vi "Tachometer.vi"(11 "Enum":enum16{"Start", "Run", "End"}(ring)) -> (3 "Tach out":dbl)   [LabVIEW 2012]
uses:
  TypeDefs/Digital Module 1.ctl
  <vilib>/Rock Robotics/SystemInterfaces/Typedef/FPGA_TypedefDigitalModule.ctl
  <vilib>/Rock Robotics/SystemInterfaces/DIO/FPGA_DIOChannel.ctl
  <vilib>/Rock Robotics/WPI/Counter/WPI_CounterDigitalInputToDigitalSource.vi
  <vilib>/Rock Robotics/WPI/Counter/WPI_CounterOpen Gear Tooth Sensor Mode.vi
panel:
  in  "Digital Module A":T1={"Module"=enum."Digital Module 1", "Unassigned"=enum."DIO 1", "Unassigned"=enum."DIO 2", "Unassigned"=enum."DIO 3", "Unassigned"=enum."DIO 4", "Unassigned"=enum."DIO 5", "Unassigned"=enum."DIO 6", "Unassigned"=enum."DIO 7", "Unassigned"=enum."DIO 8", "Unassigned"=enum."DIO 9", "Unassigned"=enum."DIO 10", "Unassigned"=enum."DIO 11", "Unassigned"=enum."DIO 12", "Unassigned"=enum."DIO 13", "Unassigned"=enum."DIO 14"}
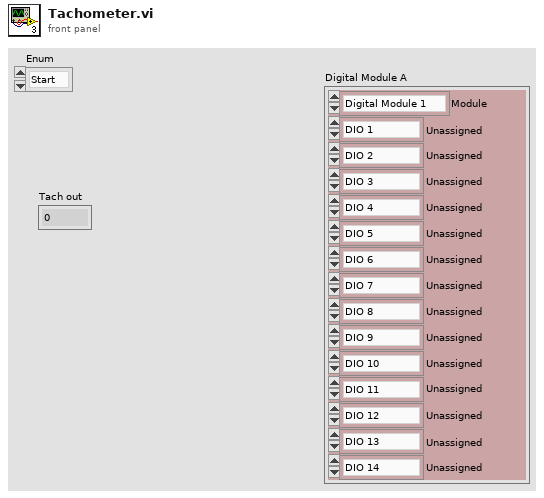
[diagram p1: front panel]
types:
  T1 = typedef "Digital Module 1.ctl" = cluster{"Module":T2, "Unassigned":T3, "Unassigned":T3, "Unassigned":T3, "Unassigned":T3, "Unassigned":T3, "Unassigned":T3, "Unassigned":T3, "Unassigned":T3, "Unassigned":T3, "Unassigned":T3, "Unassigned":T3, "Unassigned":T3, "Unassigned":T3, "Unassigned":T3}
  T2 = typedef "FPGA_TypedefDigitalModule.ctl" = enum16{"Digital Module 1", "Digital Module 2"}
  T3 = typedef "FPGA_DIOChannel.ctl" = enum8{"DIO 1", "DIO 2", "DIO 3", "DIO 4", "DIO 5", "DIO 6", "DIO 7", "DIO 8", "DIO 9", "DIO 10", "DIO 11", "DIO 12", "DIO 13", "DIO 14", "Invalid"}
  T4 = typedef "WPI_DigitalInputDevRef.ctl" = cluster{"DevStatus":errorcluster, "DIO Channel":T3, "Digital Module":T2}
  T5 = typedef "FPGA_CounterEncoderSourceConvertionLVSourceType.ctl" = cluster{"DevStatus":errorcluster, "AnalogTriggerMode?":bool, "DigitalMode":cluster{"Digital Module":T2, "DIO Channel":T6}, "AnalogTriggerMode":cluster{"AnalogTriggerIndex":T7, "OutputType":T8}}
  T6 = typedef "FPGA_DIODigitalSourceChannel.ctl" = enum8{"DIO 1", "DIO 2", "DIO 3", "DIO 4", "DIO 5", "DIO 6", "DIO 7", "DIO 8", "DIO 9", "DIO 10", "DIO 11", "DIO 12", "DIO 13", "DIO 14", "Disabled"}
  T7 = typedef "FPGA_AnalogTriggerIndex.ctl" = enum8{"Trig 0", "Trig 1", "Trig 2", "Trig 3", "Trig 4", "Trig 5", "Trig 6", "Trig 7", "Invalid"}
  T8 = typedef "FPGA_AnalogTriggerOutType.ctl" = enum16{"InWindow", "TriggerState", "Rising", "Falling"}
  T9 = typedef "WPI_CounterDevRef.ctl" = cluster{"DevStatus":errorcluster, "CntIndex":T10}
  T10 = typedef "FPGA_CounterCtrSystemIndex.ctl" = enum8{"Ctr 0", "Ctr 1", "Ctr 2", "Ctr 3", "Ctr 4", "Ctr 5", "Ctr 6", "Ctr 7", "Invalid"}
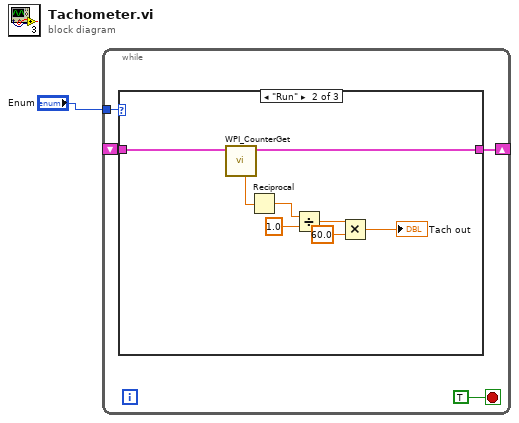
[diagram p0: block diagram]
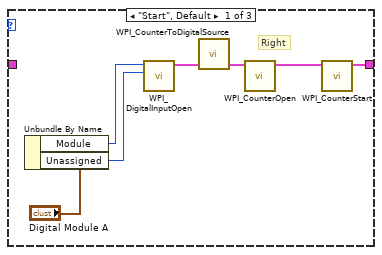
[diagram p2: hidden frame]
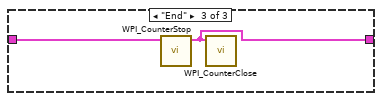
[diagram p3: hidden frame]
diagram:
  n1 = while {
    shift-right: [w4] -> _
    shift-left: _ -> [w3]
    tunnel: "Enum" -> [w2]
    stop <- TRUE stop-if-true
    n2 = case shown="\"Run\"" w2 {
      tunnel: [w8 w19 w21] -> w4
      tunnel: w3 -> [_ w20 w22]
      frame "Start", Default {
        # "Right"
        n3 = Unbundle By Name("Digital Module A") -> ("Module"=w7:T2, "Unassigned"=w6:T3)
        n4 = call <vilib>:"WPI_DigitalInputOpen.vi"("DIO Channel"=w6, "Digital Module (Module 1)"=w7) -> ("DigitalInputDevRef"=w9:T4)  [unwired: 8 in, 1 out]
        n5 = call-poly <vilib>:"WPI_CounterToDigitalSource.vi"("DigitalInputDevRef"=w9) -> ("Digital Source"=w10:T5)  [unwired: 6 in]
        n6 = call-poly <vilib>:"WPI_CounterOpen.vi"("Source"=w10) -> ("CounterDevRef"=w12:T9)  [unwired: 9 in, 1 out]
        n7 = call <vilib>:"WPI_CounterStart.vi"("CounterDevRef in"=w12) -> ("CounterDevRef out"=w8:T9)  [unwired: 9 in, 1 out]
      }
      frame "Run" {
        n8 = call <vilib>:"WPI_CounterGet.vi"("CounterDevRef in"=w20) -> ("CounterDevRef out"=w19:T9, "Period (sec)"=w17:dbl)  [unwired: 5 in, 4 out]
        n9 = Reciprocal(x=w17) -> (1/x=w16:dbl)
        n10 = Divide(x=w16, y=1.0) -> (x/y=w15:dbl)
        n11 = Multiply(x=w15, y=60.0) -> (x*y=→"Tach out":dbl)
      }
      frame "End" {
        n12 = call <vilib>:"WPI_CounterStop.vi"("CounterDevRef in"=w22) -> ("CounterDevRef out"=w21:T9)  [unwired: 9 in, 1 out]
        n13 = call <vilib>:"WPI_CounterClose.vi"("CounterDevRef"=w21) -> ()  [unwired: 10 in, 1 out]
      }
    }
  }
